vi "Read Exp_tmp.vi"(8 "error in (no error)":errorcluster, 11 "Control-Client in":refnum<class "Control-Client.lvclass">) -> (0 "error out":errorcluster, 2 "Experiment tmp":refnum<class "Experiment.lvclass">, 3 "Control-Client out":refnum<class "Control-Client.lvclass">)   [LabVIEW 2015]
uses:
  Experiments/Experiment.lvclass
  Control-Client.lvclass
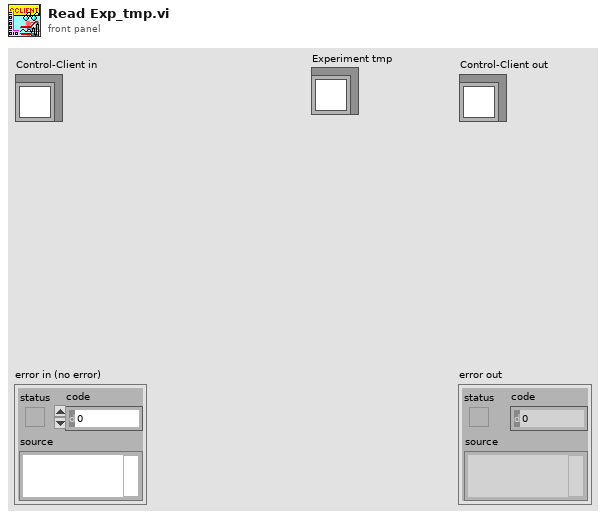
[diagram p1: front panel]
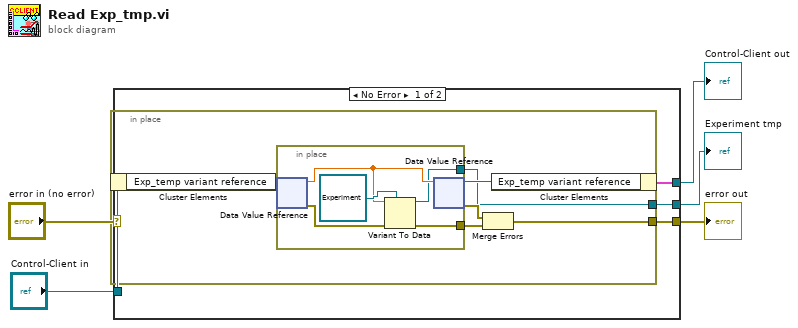
[diagram p0: block diagram]
diagram:
  n1 = case shown="No Error" "error in (no error)" {
    selector: "error in (no error)" -> [_ w21]
    tunnel: [w7 w21] -> w4
    tunnel: [w8 w22] -> w2
    tunnel: "Control-Client in" -> [w9 w22]
    tunnel: [w6 _] -> w1
    frame No Error {
      n2 = in-place {
        in-place-border: [w12] -> w7
        in-place-border: [w11] -> w6
        n3 = in-place-cluster #1(w9) -> ("Exp_temp variant reference"=w15)
        n4 = in-place {
          in-place-border: [w17] -> w11
          in-place-border: [w16] -> w10
          n5 = in-place-dvr #2(w15) -> (w18:dbl, w20:errorcluster)
          n6 = Variant To Data(error in=w20, type=refnum<class "Experiment.lvclass"> refnum ("Experiment.lvclass"), Variant=w18) -> (data=w17:refnum<class "Experiment.lvclass">, error out=w16:errorcluster)
          n7 = in-place-dvr #2(w18) -> (w14:refnum<data-value>, w13:errorcluster)
        }
        n8 = Merge Errors(w13, w10) -> (w12:errorcluster)
        n9 = in-place-cluster #1("Exp_temp variant reference"=w14) -> (w8:cluster{})
      }
    }
    frame Error {
    }
  }
  "error out" <- w4
  "Control-Client out" <- w2
  "Experiment tmp" <- w1
